vi "WPI_RobotDriveArcadeDrive_RatioCurve.vi"(7 "Sensitivity":dbl=1.0, 8 "error in (no error)":errorcluster, 9 "Y axis value (Speed)":dbl, 10 "X axis value (Curve)":dbl, 11 "RobotDriveDevRef":T1={"DevStatus"={"status"=FALSE, "code"=0, "source"=""}, "Motors[]"=[], "Square Inputs"=FALSE, "Max Output"=1.0}) -> (0 "error out":errorcluster, 2 "Motor Values":dbl[](array[numeric]), 3 "RobotDriveDevRef":T1={"DevStatus"={"status"=FALSE, "code"=0, "source"=""}, "Motors[]"=[], "Square Inputs"=FALSE, "Max Output"=1.0})   [LabVIEW 2025]
doc: "Update motors by mapping joystick axes into motor values for arcade driving. Controls the motor outputs by considering the driving speed independent of the curve rate. This VI is typically used in autonomous mode. \n\nConventions, based on HID standard, are detailed on the mapping subVI panel, but are summarized as ...\ninput of -1 means forward and left, 0 means center, 1 means back or right.\n\noutput of -1 means motor power forward, 0 means no power, and 1 means reverse.\n\nThis software is licensed. Open the labview\\readme\\WPI Robotics Library Open Source License.txt file for more information."
uses:
  <vilib>/Rock Robotics/WPI/RobotDrive/WPI_RobotDriveDevRef.ctl
  <vilib>/Rock Robotics/WPI/MotorControl/WPI_MotorControlDeviceRef.ctl
  <vilib>/Rock Robotics/WPI/MotorControl/WPI_MotorControlType.ctl
  <vilib>/Rock Robotics/SystemInterfaces/DIO/FPGA_DIOPWMChannel.ctl
  <vilib>/Rock Robotics/WPI/PWM/WPI_PWMDeadband.ctl
  <vilib>/Rock Robotics/SystemInterfaces/DIO/FPGA_DIOChannel.ctl
  <vilib>/Rock Robotics/SystemInterfaces/NetworkCommunication/NetComm_UsageReport_ResourceType.ctl
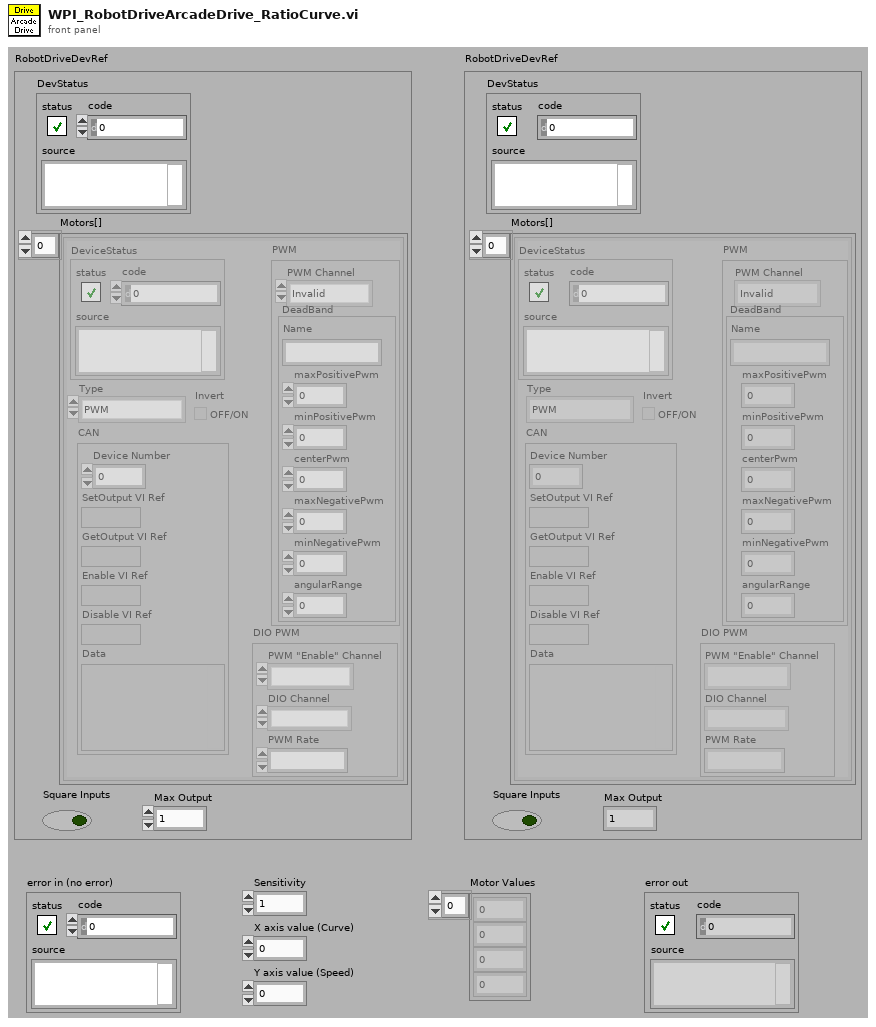
[diagram p1: front panel]
types:
  T1 = typedef "WPI_RobotDriveDevRef.ctl" = cluster{"DevStatus":errorcluster, "Motors[]":T2[], "Square Inputs":bool, "Max Output":dbl}
  T2 = typedef "WPI_MotorControlDeviceRef.ctl" = cluster{"DeviceStatus":errorcluster, "Type":T3, "PWM":cluster{"PWM Channel":T4, "DeadBand":T5}, "CAN":cluster{"Device Number":u8, "SetOutput VI Ref":variant, "GetOutput VI Ref":variant, "Enable VI Ref":variant, "Disable VI Ref":variant, "Data":variant}, "Invert":bool, "DIO PWM":cluster{"PWM \"Enable\" Channel":T4, "DIOChannel":T6, "PWM Rate":dbl}}
  T3 = typedef "WPI_MotorControlType.ctl" = enum16{"PWM", "CAN", "DIO PWM"}
  T4 = typedef "FPGA_DIOPWMChannel.ctl" = enum8{"PWM 0", "PWM 1", "PWM 2", "PWM 3", "PWM 4", "PWM 5", "PWM 6", "PWM 7", "PWM 8", "PWM 9", "PWM MXP 0", "PWM MXP 1", "PWM MXP 2", "PWM MXP 3", "PWM MXP 4", "PWM MXP 5", "PWM MXP 6", "PWM MXP 7", "PWM MXP 8", "PWM MXP 9", "Invalid"}
  T5 = typedef "WPI_PWMDeadband.ctl" = cluster{"Name":string, "maxPositivePwm":i32, "minPositivePwm":i32, "centerPwm":i32, "maxNegativePwm":i32, "minNegativePwm":i32, "angularRange":u16}
  T6 = typedef "FPGA_DIOChannel.ctl" = enum8{"DIO 0", "DIO 1", "DIO 2", "DIO 3", "DIO 4", "DIO 5", "DIO 6", "DIO 7", "DIO 8", "DIO 9", "DIO MXP 0", "DIO MXP 1", "DIO MXP 2", "DIO MXP 3", "DIO MXP 4", "DIO MXP 5", "DIO MXP 6", "DIO MXP 7", "DIO MXP 8", "DIO MXP 9", "DIO MXP 10", "DIO MXP 11", "DIO MXP 12", "DIO MXP 13", "DIO MXP 14", "DIO MXP 15", "SPI Port CS1", "SPI Port CS2", "SPI Port CS3", "SPI Port MISO", "SPI Port MOSI", "Invalid"}
  T7 = typedef "NetComm_UsageReport_ResourceType.ctl" = enum8{"Controller", "Module", "Language", "CANPlugin", "Accelerometer", "ADXL345", "AnalogChannel", "AnalogTrigger", "AnalogTriggerOutput", "CANJaguar", "Compressor", "Counter", "Dashboard", "DigitalInput", "DigitalOutput", "DriverStationCIO", "DriverStationEIO", "DriverStationLCD", "Encoder", "GearTooth", "Gyro", "I2C", "Framework", "Jaguar", "Joystick", "Kinect", "KinectStick", "PIDController", "Preferences", "PWM", "Relay", "RobotDrive", "SerialPort", "Servo", "Solenoid", "SPI", "Task", "Ultrasonic", "Victor", "Button", "Command", "AxisCamera", "PCVideoServer", "SmartDashboard", "Talon", "HiTechnicColorSensor", "HiTechnicAccel", "HiTechnicCompass", "SRF08", "AnalogOutput", "Victor SP", "Talon SRX", "CAN Talon SRX", "ADXL362 Accel", "ADXRS450 Gyro", "Rev SPARK", "Mindsensors SD540", "Digital Filter", "ADIS16448", "PDP", "PCM", "PigeonIMU", "Nidec Brushless", "CTRE CANifier", "CTRE TalonFX", "CTRE Future 1", "CTRE Future 2", "CTRE Future 3", "CTRE Future 4", "CTRE Future 5", "CTRE Future 6", "Linear Filter", "Xbox Controller", "USB Camera", "NavX", "Pixy", "Pixy2", "ScanseSweep", "Shuffleboard", "CAN", "Digilent DMC60", "PWM Victor SPX", "Rev SPARK MAX PWM", "Rev SPARK MAX CAN", "ADIS16470", "PIDController2", "ProfiledPIDController", "Kinematics", "Odometry", "Units", "Trapezoid Profile", "DutyCycle", "Addressable LEDs", "Fusion Venom", "CTRE Future 7", "CTRE Future 8", "CTRE Future 9", "CTRE Future 10", "CTRE Future 11", "CTRE Future 12", "CTRE Future 13", "CTRE Future 14", "Exponential Profile", "PS4 Controller", "Photon Camera", "Photon Pose Estimator", "Path Planner Path", "Path Planner Auto", "Path Finding Command", "Redux Future 1", "Redux Future 2", "Redux Future 3", "Redux Future 4", "Redux Future 5", "Rev SPARK Flex CAN", "Rev SPARK Flex PWM", "LEDPattern", "LinearQuadraticRegulator", "KalmanFilter", "PoseEstimator", "PoseEstimator3d", "LinearSystemLoop", "WPILib_future7", "WPILib_future8", "Rev_ServoHub", "YAMS", "LumenLabs_ConnectorX", "LumenLabs_ConnectorXLED"}
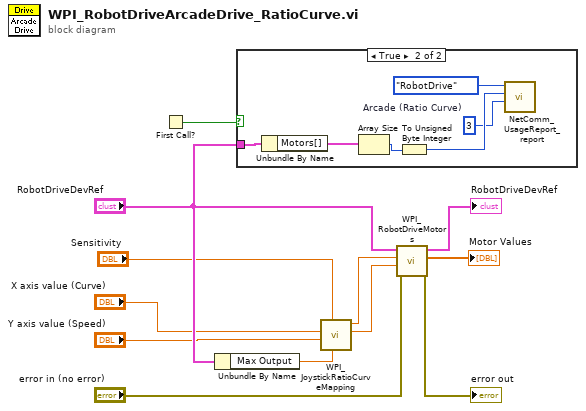
[diagram p0: block diagram]
diagram:
  n1 = First Call?() -> (First Call?: T/F=w9:bool)
  n2 = Unbundle By Name("RobotDriveDevRef") -> ("Max Output"=w4:dbl)
  n3 = case shown="True" w9 {
    tunnel: "RobotDriveDevRef" -> [_ w13]
    frame False {
    }
    frame True {
      w16 = u8 3  # Arcade (Ratio Curve)
      n4 = Unbundle By Name(w13) -> ("Motors[]"=w15:T2[])
      n5 = Array Size(array=w15) -> (size(s)=w14:i32)
      n6 = To Unsigned Byte Integer(number=w14) -> (unsigned 8bit integer=w17:u8)
      n7 = call <vilib>:"NetComm_UsageReport_report.vi"("Context"=w16, "Instance Number"=w17, "Resource Type"=NetComm_UsageReport_ResourceType."RobotDrive") -> ()  [unwired: 9 in]
    }
  }
  n8 = call <vilib>:"WPI_JoystickRatioCurveMapping.vi"("Max Output"=w4, "Sensitivity"="Sensitivity", "Y axis value (Speed)"="Y axis value (Speed)", "X axis value (Curve)"="X axis value (Curve)") -> ("Right Motor Value"=w11:dbl, "Left Motor Value"=w12:dbl)  [unwired: 6 in]
  n9 = call <vilib>:"WPI_RobotDriveMotors.vi"("error in (no error)"="error in (no error)", "RightSpeed"=w11, "LeftSpeed"=w12, "RobotDriveDevRef"="RobotDriveDevRef") -> ("error out"=→"error out":errorcluster, "Motor Values"=→"Motor Values":dbl[], "RobotDriveDevRef"=→"RobotDriveDevRef":T1)  [unwired: 5 out]
